vi "Service Request Enable.vi"(0 "VISA resource name":refnum<visa-resource-name>, 5 "Service Request Enable":T1, 11 "error in (no error)":errorcluster) -> (4 "VISA resource name out":refnum<visa-resource-name>, 15 "error out":errorcluster)   [LabVIEW 2020, in "eec EST 300.lvlib"]
doc: "Service Request enable register controls which bits from the Status Byte should be used to generate a service request when the bit value = 1.\n\nThe Standard Event Register consists of the following 8 bits.\nBit 0: MSB = Measurement Summary Bit\nBit 1: not used\nBit 2: EAV = Error Available \nBit 3: QSB = Questionable Summary Bit\nBit 4: MAV = Message Available\nBit 5: ESB = Event Summary Bit \nBit 6: not used\nBit 7: OSB = Operation Summary Bit\n\nExample:\n\nIf the user wants to generate SRQ(Service Request) when there is MAV and EAV only the binary mask (00000101|bin=5|dec) should be used."
uses:
  <instrlib>/eec EST 300/eec EST 300.lvlib
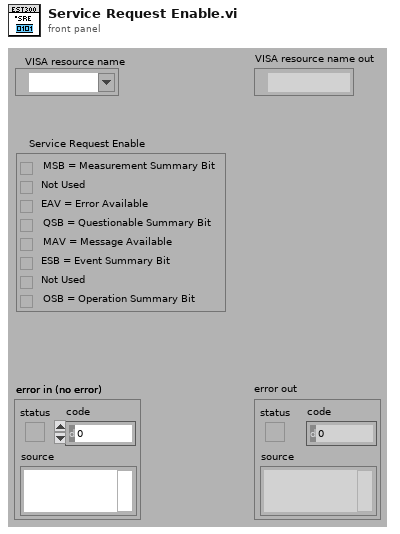
[diagram p1: front panel]
types:
  T1 = cluster{"MSB = Measurement Summary Bit":bool, "Not Used":bool, "EAV = Error Available":bool, "QSB = Questionable Summary Bit":bool, "MAV = Message Available":bool, "ESB = Event Summary Bit":bool, "Not Used":bool, "OSB = Operation Summary Bit":bool}
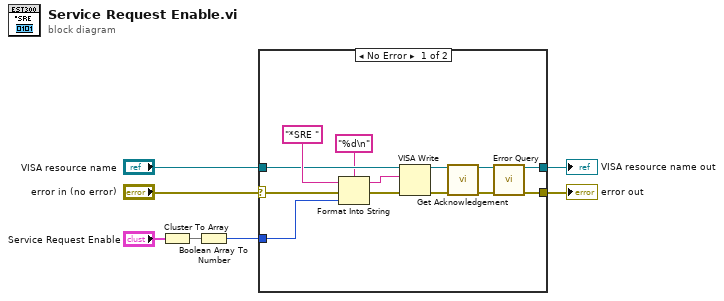
[diagram p0: block diagram]
diagram:
  n1 = Cluster To Array(cluster="Service Request Enable") -> (array=w3:bool[])
  n2 = Boolean Array To Number(Boolean array=w3) -> (number=w1:u32)
  n3 = case shown="No Error" "error in (no error)" {
    selector: "error in (no error)" -> [w16 w21]
    tunnel: w1 -> [w20 _]
    tunnel: "VISA resource name" -> [w15 w22]
    tunnel: [w14 w22] -> w4
    tunnel: [w13 w21] -> w5
    frame No Error {
      n4 = Format Into String(format string="%d\n", initial string="*SRE " ("Command to Send"), error in=w16, w20) -> (resulting string=w18:string, error out=w17:errorcluster)
      n5 = VISA Write(VISA resource name=w15, write buffer=w18, error in (no error)=w17) -> (VISA resource name out=w9:refnum<visa-resource-name>, error out=w8:errorcluster)  [unwired: 1 out]
      n6 = call <instrlib>:"Get Acknowledgement.vi"("VISA resource name"=w9, "error in (no error)"=w8) -> ("VISA resource name out"=w10:refnum<visa-resource-name>, "error out"=w11:errorcluster)  [unwired: 12 in]
      n7 = call <instrlib>:"Error Query.vi"("VISA resource name"=w10, "error in (no error)"=w11) -> ("VISA resource name out"=w14:refnum<visa-resource-name>, "error out"=w13:errorcluster)  [unwired: 10 in, 2 out]
    }
    frame Error {
    }
  }
  "error out" <- w5
  "VISA resource name out" <- w4
